vi "EF_FeatureExtraction.vi"(8 "error in (no error)":errorcluster, 10 "FeatureExtractionParams":T2={"FeatureExtractionMethod"=enum."Amplitude Variance", "Parameter #1"=0.5, "Parameter #2"=15.0} {"Parameter #2" min=0.0 max=256.0 step=0.1; "Parameter #1" min=0.0 max=256.0 step=0.1}, 11 "Array Of Waveforms in":waveform(dbl)[](array[waveform])) -> (0 "error out (no error)":errorcluster, 1 "FeatureVector Length":i32, 2 "FeatureVector":dbl[](array[numeric]), 3 "Feature Matrix":dbl[][](array[numeric]))   [LabVIEW 2016, in "Feature Extraction.lvlib"]
uses:
  Feature Extraction.lvlib
  EF_FeatureExtractionMethods.ctl
panel:
  # "This VI is a part of BCI Design library, http://www.ru-bci.org \nCopyright © 2020, Sotnikov Peter, All rights reserved. License: GNU GPLv3"
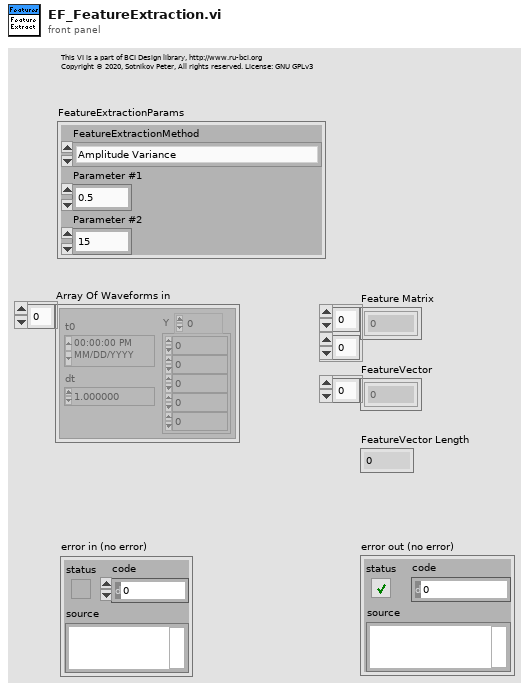
[diagram p1: front panel]
types:
  T1 = typedef "Feature Extraction.lvlib/EF_FeatureExtractionMethods.ctl" = enum16{"Amplitude Variance", "Amplitude Entropy", "EEG Spectrum (FourierTransform)", "EEG Spectrum (WaveletTransform)", "Spectral Power of EEG Rhythms (FourierTransform)", "Spectral Power of EEG Rhythms (WaveletTransform)", "Wavelet Scalogram", "Signal Downsampling", "Vector Autoregressive Model", "EEG Bicoherence"}
  T2 = cluster{"FeatureExtractionMethod":T1, "Parameter #1":dbl, "Parameter #2":dbl}
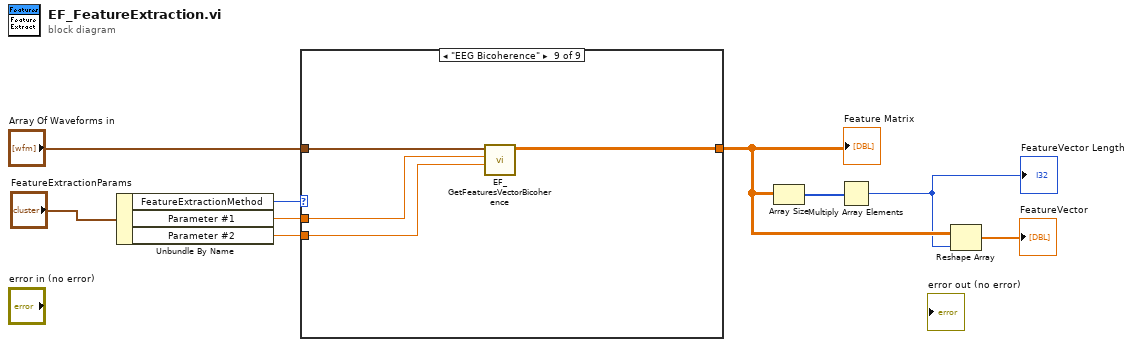
[diagram p0: block diagram]
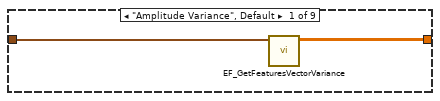
[diagram p2: hidden frame]
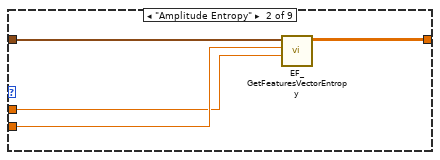
[diagram p3: hidden frame]
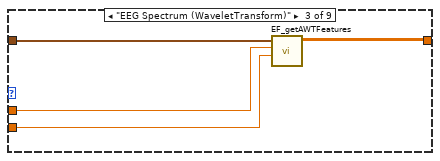
[diagram p4: hidden frame]
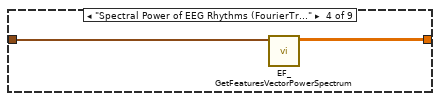
[diagram p5: hidden frame]
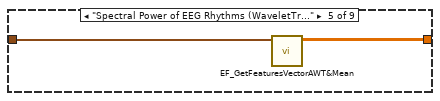
[diagram p6: hidden frame]
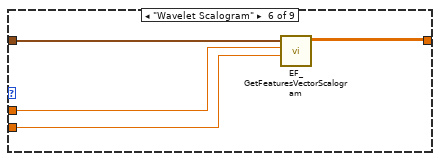
[diagram p7: hidden frame]
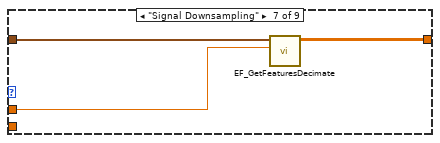
[diagram p8: hidden frame]
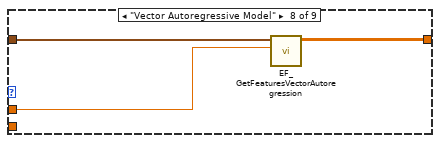
[diagram p9: hidden frame]
diagram:
  n1 = Unbundle By Name("FeatureExtractionParams") -> ("FeatureExtractionMethod"=w9:T1, "Parameter #1"=w3:dbl, "Parameter #2"=w1:dbl)
  n2 = case shown="\"EEG Bicoherence\"" w9 {
    tunnel: "Array Of Waveforms in" -> [w11 w15 w19 w21 w23 w27 w30 w33 w37]
    tunnel: [w10 w14 w18 w20 w22 w26 w29 w32 w34] -> w7
    tunnel: w3 -> [_ w12 w17 _ _ w25 w28 w31 w36]
    tunnel: w1 -> [_ w13 w16 _ _ w24 _ _ w35]
    frame "Amplitude Variance", Default {
      n3 = call "EF_GetFeaturesVectorVariance.vi"("Array Of Waveforms in"=w11) -> ("Features Array out"=w10:dbl[][])  [unwired: 9 in, 1 out]
    }
    frame "Amplitude Entropy" {
      n4 = call "EF_GetFeaturesVectorEntropy.vi"("Amplitude Min"=w12, "Amplitude Max"=w13, "Array Of Waveforms in"=w15) -> ("Features Array out"=w14:dbl[][])  [unwired: 7 in, 1 out]
    }
    frame "EEG Spectrum (WaveletTransform)" {
      n5 = call "EF_getAWTFeatures.vi"("High cutoff frequency"=w16, "Low cutoff frequency"=w17, "Array Of Waveforms in"=w19) -> ("MatrixOfMeanPowers"=w18:dbl[][])  [unwired: 7 in, 1 out]
    }
    frame "Spectral Power of EEG Rhythms (FourierTransform)" {
      n6 = call "EF_GetFeaturesVectorPowerSpectrum.vi"("Array Of Waveforms in"=w21) -> ("Features Array out"=w20:dbl[][])  [unwired: 9 in, 1 out]
    }
    frame "Spectral Power of EEG Rhythms (WaveletTransform)" {
      n7 = call "EF_GetFeaturesVectorAWT&Mean.vi"("Array Of Waveforms in"=w23) -> ("Features Array out"=w22:dbl[][])  [unwired: 9 in, 1 out]
    }
    frame "Wavelet Scalogram" {
      n8 = call "EF_GetFeaturesVectorScalogram.vi"("High cutoff frequency"=w24, "Low cutoff frequency"=w25, "Array Of Waveforms in"=w27) -> ("StackedScalograms"=w26:dbl[][])  [unwired: 6 in, 2 out]
    }
    frame "Signal Downsampling" {
      n9 = call "EF_GetFeaturesDecimate.vi"("Decimating Factor"=w28, "Array Of Waveforms in"=w30) -> ("Features Array out"=w29:dbl[][])  [unwired: 8 in, 1 out]
    }
    frame "Vector Autoregressive Model" {
      n10 = call "EF_GetFeaturesVectorAutoregression.vi"("AR order"=w31, "Array Of Waveforms in"=w33) -> ("Features Array out"=w32:dbl[][])  [unwired: 8 in, 1 out]
    }
    frame "EEG Bicoherence" {
      n11 = call "EF_GetFeaturesVectorBicoherence.vi"("High cutoff frequency"=w35, "Low cutoff frequency"=w36, "Array Of Waveforms in"=w37) -> ("Bicoherence features out"=w34:dbl[][])  [unwired: 7 in, 1 out]
    }
  }
  "Feature Matrix" <- w7
  n12 = Array Size(array=w7) -> (size(s)=w5:i32[])
  n13 = Multiply Array Elements(1:w5) -> (0:w4:i32)
  "FeatureVector Length" <- w4
  n14 = Reshape Array(w7, w4) -> (→"FeatureVector":dbl[])
